vi "EXAMPLE_APPLICATION.vi"() -> ()   [LabVIEW 2014]
uses:
  DEF-SineSettings.ctl
  TagDB/_Support/Access/_setAnything.vi
  TagDB/_Support/Properties/tagDB dbChanged.vi
  TagDB/_Support/Access/_variant.vi
  TagDB/_Support/Error/_[error50002]Invalid DataType.vi
  TagDB/_XNode/tagDB_setValue.xnode/tagDB_setValue.xnode
  TagDB/tagDB_Def.ctl
  TagDB/_XNode/tagDB_value.xnode/tagDB_value.xnode
  TagDB/TagDB(dev).lvlib
panel:
  in  "Model":bool
  out "Sine Settings":T1={"frequency"=10.0, "amplitude"=1.0, "phase"=0.0, "sampling info"={"Fs"=1000.0, "#s"=1000.0}} {"frequency" format="%0.2p"; "amplitude" format="%0.2p"; "phase" format="%.2p"; "sampling info"."Fs" format="%.2p"}
  out "Waveform Graph":waveform(dbl)(graph)
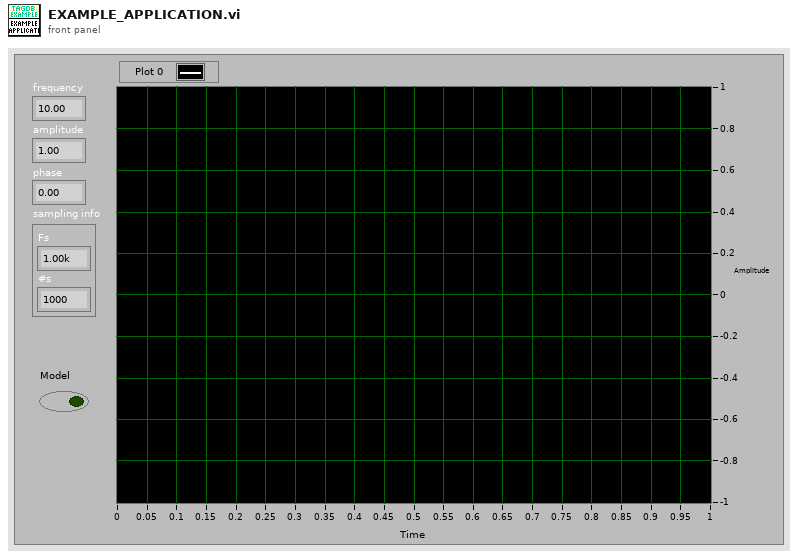
[diagram p1: front panel]
types:
  T1 = typedef "DEF-SineSettings.ctl" = cluster{"frequency":dbl, "amplitude":dbl, "phase":dbl, "sampling info":cluster{"Fs":dbl, "#s":dbl}}
  T2 = typedef "TagDB(dev).lvlib/tagDB_Def.ctl" = refnum<k1>
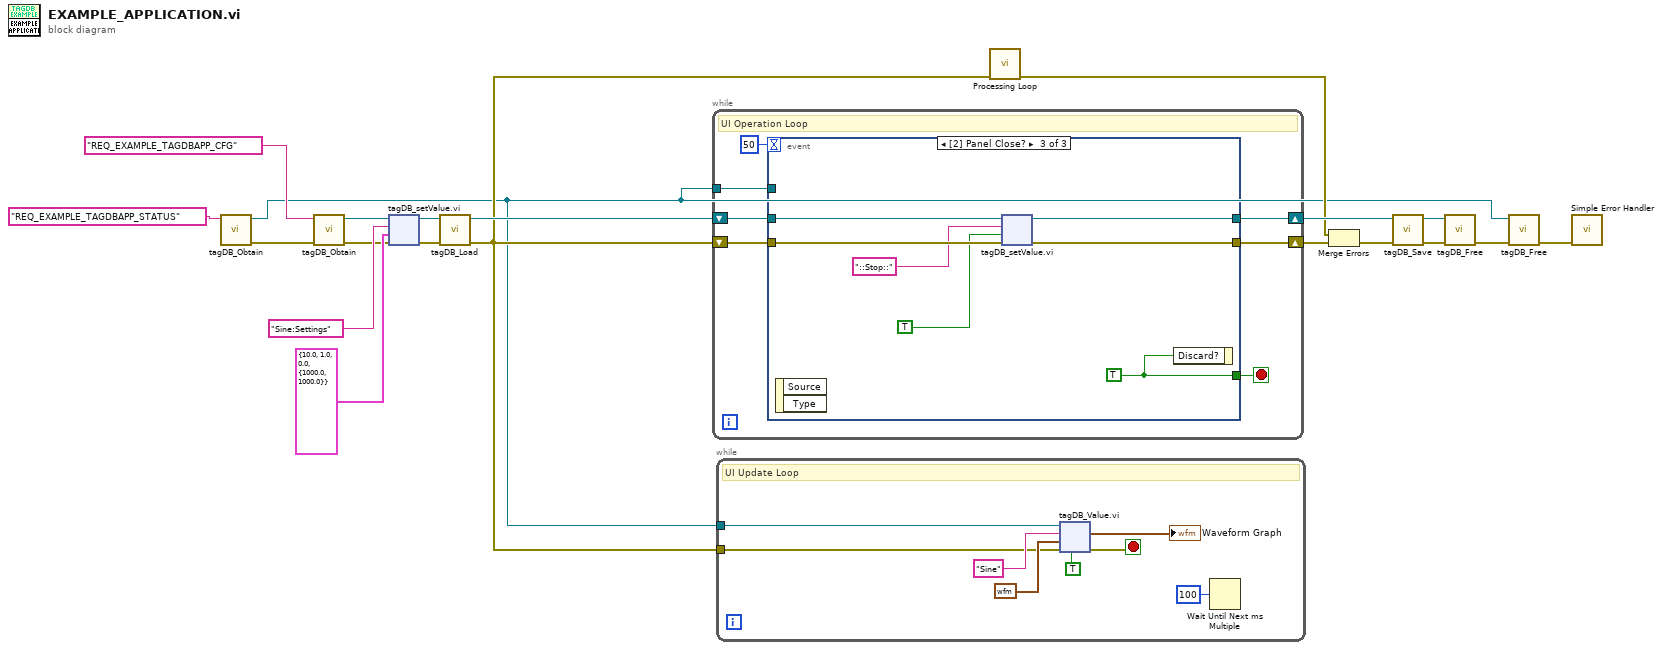
[diagram p0: block diagram]
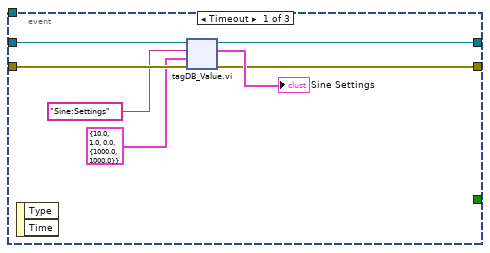
[diagram p2: hidden frame]
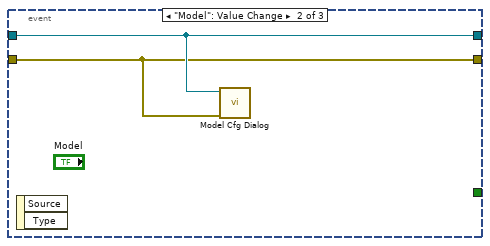
[diagram p3: hidden frame]
diagram:
  n1 = call "tagDB_Obtain.vi"("name (unnamed)"="REQ_EXAMPLE_TAGDBAPP_STATUS") -> ("error out"=w14:errorcluster, "DB"=w1:T2)  [unwired: 4 in, 1 out]
  n2 = call "tagDB_Obtain.vi"("error in (no error)"=w14, "name (unnamed)"="REQ_EXAMPLE_TAGDBAPP_CFG") -> ("error out"=w2:errorcluster, "DB"=w3:T2)  [unwired: 3 in, 1 out]
  n3 = xnode "tagDB_setValue.vi"("DB Ref"=w3, "name"="Sine:Settings", "value"=T1 {"frequency"=10.0, "amplitude"=1.0, "phase"=0.0, "sampling info"={"Fs"=1000.0, "#s"=1000.0}} ("Sine Settings"), "Error In"=w2) -> ("DB Ref(dup)"=w7:T2, "Error Out"=w6:errorcluster)  [unwired: 1 out]
  n4 = call "tagDB_Load.vi"("error in (no error)"=w6, "DB Ref"=w7) -> ("error out"=w10:errorcluster, "DB Ref(dup)"=w11:T2)  [unwired: 8 in]
  n5 = while {
    shift-right: [w24] -> w17
    shift-left: w11 -> [w25]
    shift-right: [w23] -> w16
    shift-left: w10 -> [w22]
    tunnel: w1 -> [w21]
    stop <- w27 stop-if-true
    # "UI Operation Loop"
    n6 = event shown="[2] Panel Close?" {
      selector: _ -> [_ _ _]
      dyn-events: _ -> [_ _ _]
      timeout: 50 -> [_ _ _]
      tunnel: [_ _ w88] -> w27
      tunnel: w25 -> [w34 w81 w87]
      tunnel: [w32 w81 w86] -> w24
      tunnel: [w28 w80 w84] -> w23
      tunnel: w22 -> [w33 w80 w85]
      tunnel: w21 -> [_ _ _]
      event Timeout {
        n7 = event-data() -> ()  [unwired: 1 in, 2 out]
        n8 = xnode "tagDB_Value.vi"("error in (no error)"=w33, "DB Ref"=w34, "Type"=T1 {"frequency"=10.0, "amplitude"=1.0, "phase"=0.0, "sampling info"={"Fs"=1000.0, "#s"=1000.0}} ("Sine Settings"), "name"="Sine:Settings") -> ("error out"=w28:errorcluster, "DB Ref(dup)"=w32:T2, "value"=→"Sine Settings":T1)  [unwired: 1 in]
      }
      event "Model": Value Change {
        n9 = event-data() -> ()  [unwired: 1 in, 2 out]
        n10 = call "Model Cfg Dialog.vi"("error in (no error)"=w80, "DB Ref"=w81) -> ()  [unwired: 9 in, 1 out]
      }
      event Panel Close? {
        w88 = TRUE
        n11 = event-data() -> ()  [unwired: 1 in, 2 out]
        n12 = xnode "tagDB_setValue.vi"("DB Ref"=w87, "name"="::Stop::", "value"=TRUE, "Error In"=w85) -> ("DB Ref(dup)"=w86:T2, "Error Out"=w84:errorcluster)  [unwired: 1 out]
        n13 = event-data ("Event Filter Node")("Discard?"=w88) -> ()  [unwired: 1 in, 1 out]
      }
    }
  }
  n14 = while {
    tunnel: w1 -> [w103]
    tunnel: w10 -> [w98]
    stop <- w102 stop-if-true
    # "UI Update Loop"
    n15 = xnode "tagDB_Value.vi"("error in (no error)"=w98, "DB Ref"=w103, "Type"=waveform(dbl) {"t0"=timestamp(0 s since 1904-01-01), "dt"=1.0, "Y"=[]} ("signal out"), "Add wih NonExist?"=TRUE, "name"="Sine") -> ("error out"=w102:errorcluster, "value"=→"Waveform Graph":waveform(dbl))  [unwired: 1 out]
    n16 = Wait Until Next ms Multiple(millisecond multiple=u32 100 ("milliseconds to wait")) -> ()  [unwired: 1 out]
  }
  n17 = call "Processing Loop.vi"("error in (no error)"=w10) -> ("error out"=w8:errorcluster)  [unwired: 10 in]
  n18 = Merge Errors(w8, w16) -> (w9:errorcluster)
  n19 = call "tagDB_Save.vi"("error in (no error)"=w9, "DB Ref"=w17) -> ("error out"=w18:errorcluster, "DB Ref(dup)"=w19:T2)  [unwired: 8 in]
  n20 = call "tagDB_Free.vi"("error in (no error)"=w18, "DB Ref"=w19) -> ("error out"=w13:errorcluster)  [unwired: 9 in]
  n21 = call "tagDB_Free.vi"("error in (no error)"=w13, "DB Ref"=w1) -> ("error out"=w12:errorcluster)  [unwired: 9 in]
  n22 = call <vilib>:"Simple Error Handler.vi"("error in (no error)"=w12) -> ()  [unwired: 4 in, 5 out]
